vi "Sort 2D Array.vi"(0 "Sort By (Column:F)":bool, 1 "Order (Ascending:F)":bool, 2 "Unsorted 2D Array":dbl[][](array[numeric]) format="%.2f", 3 "Column/Row to Sort By":u32, 4 "Secondary Column/Row to Sort By (-1 for None)":i32=-1) -> (5 "Sorted 2D Array":dbl[][](array[numeric]) format="%.2f", 6 "Index Out of Range?":bool)   [LabVIEW 2020]
doc: "This VI sorts a 2D array of any size in descending or ascending order based on a column or row whose index you specify. It does not use a secondary column/row to sort by. So, if the main column or row has multiple elements that have the same value, the first of those elements that is found in the original array is going to be the element placed first in the sorted array. To use, enter an array in the 2D Array and select whether to sort by Ascending or Descending order and whether to sort based on a column or row and the index of that column or row. This VI can also be used as a SubVI and the Values can be passed to it."
panel:
  # "This VI sorts a 2D array of any size in descending or ascending order based on a column or row whose index you specify. It does not use a secondary column/row to sort by. So, if the main column or row has multiple elements that have the same value, the first of those elements that is found in the original array is going to be the element placed first in the sorted array. To use, enter an array in the 2D Array and select whether to sort by Ascending or Descending order and whether to sort based on a column or row and the index of that column or row. This VI can also be used as a SubVI and the Values can be passed to it."
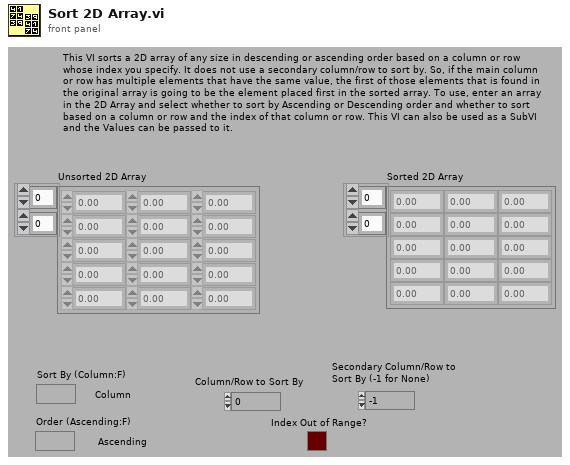
[diagram p1: front panel]
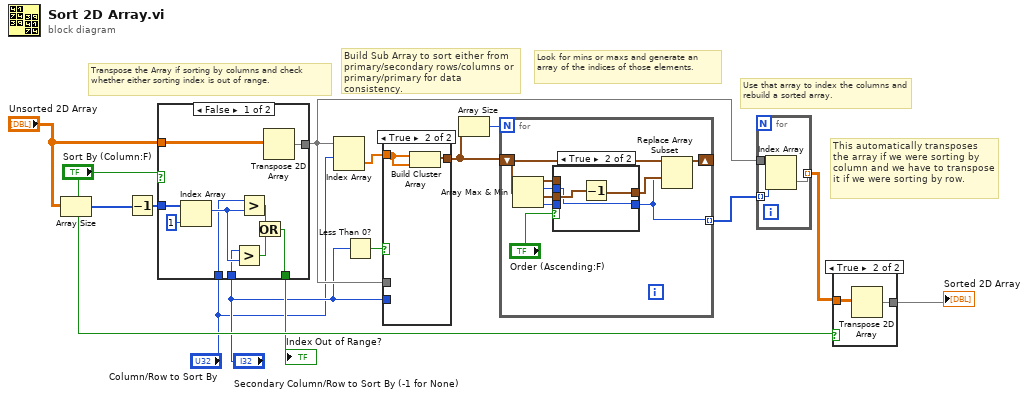
[diagram p0: block diagram]
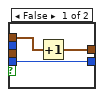
[diagram p3: hidden frame]
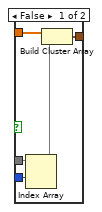
[diagram p4: hidden frame]
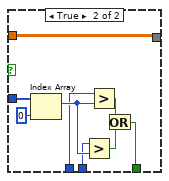
[diagram p5: hidden frame]
diagram:
  # "This automatically transposes the array if we were sorting by column and we have to transpose it if we were sorting by row."
  # "Use that array to index the columns and rebuild a sorted array."
  # "Look for mins or maxs and generate an array of the indices of those elements."
  # "Build Sub Array to sort either from primary/secondary rows/columns or primary/primary for data consistency."
  # "Transpose the Array if sorting by columns and check whether either sorting index is out of range."
  n1 = Array Size(array="Unsorted 2D Array") -> (size(s)=w7:i32[])
  n2 = Decrement(x=w7) -> (x-1=w3:i32[])
  n3 = case shown="False" "Sort By (Column:F)" {
    tunnel: "Unsorted 2D Array" -> [w25 w34]
    tunnel: [w24 w34] -> w11
    tunnel: w3 -> [w23 w29]
    tunnel: [w18 w28] -> w6
    tunnel: "Secondary Column/Row to Sort By (-1 for None)" -> [w16 w27]
    tunnel: "Column/Row to Sort By" -> [w17 w26]
    frame False {
      n4 = Index Array(array=w23, index=1 ("Index")) -> (element=w21:i32)
      n5 = Greater?(x=w16, y=w21) -> (0:w19:bool)
      n6 = Greater?(x=w17, y=w21) -> (0:w20:bool)
      n7 = Or(x=w20, y=w19) -> (x .or. y?=w18:bool)
      n8 = Transpose 2D Array(2D array=w25) -> (transposed array=w24:dbl[][])
    }
    frame True {
      n9 = Index Array(array=w29, index=0 ("Index")) -> (element=w31:i32)
      n10 = Greater?(x=w27, y=w31) -> (0:w33:bool)
      n11 = Greater?(x=w26, y=w31) -> (0:w32:bool)
      n12 = Or(x=w32, y=w33) -> (x .or. y?=w28:bool)
    }
  }
  "Index Out of Range?" <- w6
  n13 = Index Array(array=w11, index (row)="Column/Row to Sort By") -> (element=w14:dbl[])  [unwired: 1 in]
  n14 = Less Than 0?(x="Secondary Column/Row to Sort By (-1 for None)") -> (x < 0?=w15:bool)
  n15 = case shown="True" w15 {
    tunnel: w14 -> [w37 w40]
    tunnel: w11 -> [w39 _]
    tunnel: "Secondary Column/Row to Sort By (-1 for None)" -> [w38 _]
    tunnel: [w35 w41] -> w13
    frame False {
      n16 = Index Array(array=w39, index (row)=w38) -> (element=w36:dbl[])  [unwired: 1 in]
      n17 = Build Cluster Array(w37, w36) -> (w35:cluster{"Numeric":dbl, "Numeric":dbl}[])
    }
    frame True {
      n18 = Build Cluster Array(w40, w40) -> (w41:cluster{"Numeric":dbl, "Numeric":dbl}[])
    }
  }
  n19 = Array Size(array=w13) -> (size(s)=w12:i32)
  n20 = for {
    N: w12 -> [_]
    shift-right: [w49] -> _
    shift-left: w13 -> [w50]
    tunnel: [w43] -> w9 mode=indexing
    n21 = Array Max & Min(array=w50) -> (max value=w45:cluster{"Numeric":dbl, "Numeric":dbl}, max index (indices)=w46:i32, min value=w47:cluster{"Numeric":dbl, "Numeric":dbl}, min index (indices)=w48:i32)
    n22 = case shown="True" "Order (Ascending:F)" {
      tunnel: w48 -> [w51 _]
      tunnel: w47 -> [_ w56]
      tunnel: w46 -> [_ w54]
      tunnel: w45 -> [w53 _]
      tunnel: [w52 w55] -> w44
      tunnel: [w51 w54] -> w43
      frame False {
        n23 = Increment(x=w53) -> (x+1=w52:cluster{"Numeric":dbl, "Numeric":dbl})
      }
      frame True {
        n24 = Decrement(x=w56) -> (x-1=w55:cluster{"Numeric":dbl, "Numeric":dbl})
      }
    }
    n25 = Replace Array Subset(array=w50, new element=w44, index=w43) -> (w49:cluster{"Numeric":dbl, "Numeric":dbl}[])
  }
  n26 = for {
    tunnel: w9 -> [w59] mode=indexing
    tunnel: w11 -> [w58]
    tunnel: [w57] -> w10 mode=indexing
    n27 = Index Array(array=w58, index (col)=w59) -> (element=w57:dbl[])  [unwired: 1 in]
  }
  n28 = case shown="True" "Sort By (Column:F)" {
    tunnel: w10 -> [w60 w62]
    tunnel: [w60 w61] -> w1
    frame False {
    }
    frame True {
      n29 = Transpose 2D Array(2D array=w62) -> (transposed array=w61:dbl[][])
    }
  }
  "Sorted 2D Array" <- w1
